vi "GSwFormDSP_Create.vi"(0 "reference in":refnum<class "GSwFormDSP.lvclass">, 5 "error in (no error)":errorcluster, 7 "Application Name":string, 9 "State Queue":string[](array[string])) -> (14 "reference out":refnum<class "GSwFormDSP.lvclass">, 19 "error out":errorcluster)   [LabVIEW 2020, in "GSwFormDSP.lvclass"]
doc: "Constructor."
uses:
  GSwFormDSP.lvclass
  C:/Program Files/National Instruments/LabVIEW 2020/vi.lib/addons/_AddQ/G#Object/G#Object.lvclass
  C:/Users/fcharett/docsWork/coding/20SPWB/C/Users/fcharett/docsWork/coding/LabVIEW/API/Generic Utilities_class/Generic Utilities.lvclass
  functions/TDF Parameters.ctl
  <vilib>/addons/_AddQ/G#Object/G#Object.lvclass
  Generic Utilities_class/Generic Utilities.lvclass
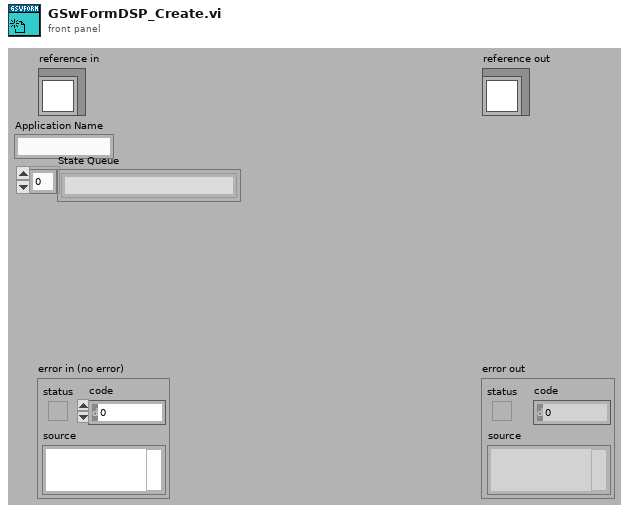
[diagram p1: front panel]
types:
  T1 = typedef "GSwFormDSP.lvclass/TDF Parameters.ctl" = cluster{"Filter":enum32{"Lowpass", "Highpass", "Bandpass", "Bandstop"}, "Type:":enum16{"Butterworth", "Chebyshev", "Inv Chebyshev", "Elliptic", "Bessel"}, "LP cutoff freq":dbl, "HP cutoff freq":dbl, "Order":i32, "passband ripple (dB)":dbl, "stopband attenuation (dB)":dbl, "Phaseless Filter":bool, "Include Fade IN and OUT":bool}
  T2 = typedef "GSwFormDSP.lvclass/ObjectAttributesRef.ctl" = refnum<data-value>
  T3 = typedef "GSwFormDSP.lvclass/ObjectAttributes.ctl" = cluster{"Wform Ref":refnum<data-value>, "Nb Signals":i32, "Spectral Function Parameters":T4, "FFT":waveform(cdb)[], "Nb FFT":i32, "Nb Averages":i32[], "Reference Indexes":i32[], "Response Indexes":i32[], "Coherence":waveform(dbl)[], "TDF Parameters":T1, "DAQ":cluster{"Duration (sec)":dbl, "Buffer Size (Samples)":i32, "Offset (Samples)":i32}, "Filter Impulse Response (TDF)":waveform(dbl), "Sound Playback":T6}
  T4 = typedef "GSwFormDSP.lvclass/Spectral Parameters.ctl" = cluster{"Frequency resolution (Hz)":dbl, "Overlap":dbl, "Window":T5}
  T5 = typedef "NI_AALPro.lvlib/windowTd.ctl" = u32
  T6 = typedef "GSwFormDSP.lvclass/Sound Playback.ctl" = cluster{"Timer start (ms)":u32, "task ID":T7, "Cursor Init Location (s)":dbl, "SC Volume":dbl}
  T7 = typedef "Sound Output Task ID.ctl" = u32
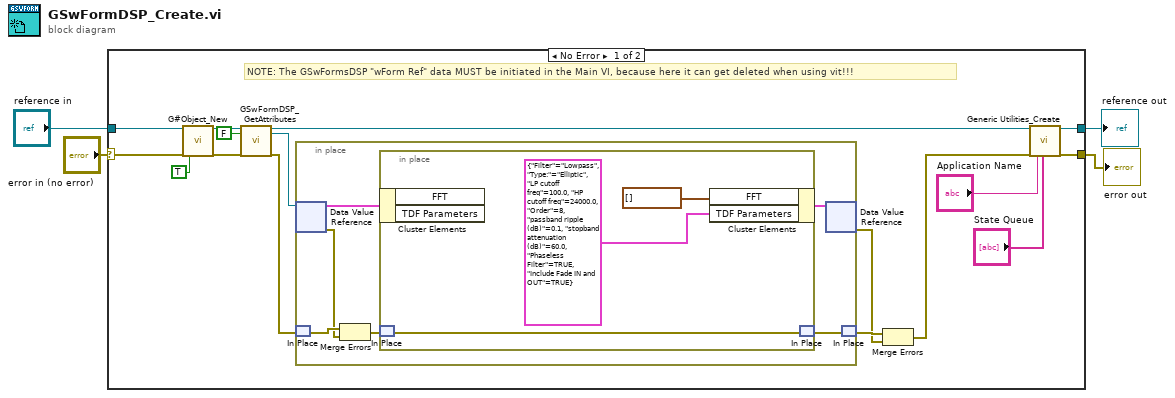
[diagram p0: block diagram]
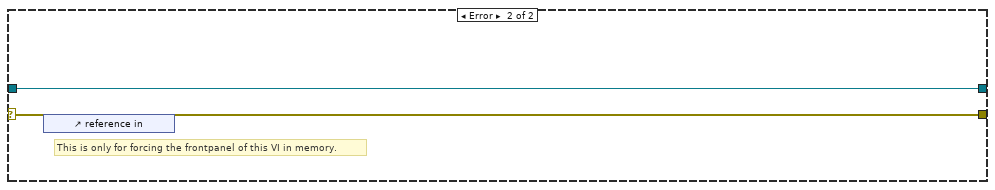
[diagram p2: hidden frame]
diagram:
  n1 = case shown="No Error" "error in (no error)" {
    selector: "error in (no error)" -> [w8 w31]
    tunnel: [w14 w31] -> w3
    tunnel: [w13 w30] -> w1
    tunnel: "reference in" -> [w7 w30]
    frame No Error {
      # "NOTE: The GSwFormsDSP \"wForm Ref\" data MUST be initiated in the Main VI, because here it can get deleted when using vit!!!"
      n2 = call <vilib>:"G#Object_New.vi"("reference in"=w7, "error in (no error)"=w8, "user counter (T)?"=TRUE ("User Counter")) -> ("reference out"=w19:refnum<class "GSwFormDSP.lvclass">, "error out"=w18:errorcluster)  [unwired: 14 in, 1 out]
      n3 = call "GSwFormDSP_GetAttributes.vi"("reference in"=w19, "return data? (T)"=FALSE, "error in (no error)"=w18) -> ("reference out"=w9:refnum<class "GSwFormDSP.lvclass">, "attributes ref"=w16:T2, "error out"=w12:errorcluster)  [unwired: 13 in, 1 out]
      n4 = in-place {
        n5 = in-place-dvr #1(w16) -> (w25:T3, w23:errorcluster)
        n6 = in-place-match #2(w12) -> (w24:errorcluster)
        n7 = Merge Errors(w24, w23) -> (w22:errorcluster)
        n8 = in-place {
          n9 = in-place-cluster #3(w25) -> ()  [unwired: 2 out]
          n10 = in-place-match #4(w22) -> (w27:errorcluster)
          n11 = in-place-cluster #3("FFT"=waveform(cdb)[] [], "TDF Parameters"=T1 {"Filter"=enum."Lowpass", "Type:"=enum."Elliptic", "LP cutoff freq"=100.0, "HP cutoff freq"=24000.0, "Order"=8, "passband ripple (dB)"=0.1, "stopband attenuation (dB)"=60.0, "Phaseless Filter"=TRUE, "Include Fade IN and OUT"=TRUE}) -> (w26:T3)
          n12 = in-place-match #4(w27) -> (w21:errorcluster)
        }
        n13 = in-place-dvr #1(w26) -> (w10:errorcluster)  [unwired: 1 out]
        n14 = in-place-match #2(w21) -> (w11:errorcluster)
      }
      n15 = Merge Errors(w11, w10) -> (w15:errorcluster)
      n16 = call "Generic Utilities_Create.vi"("reference in"=w9, "error in (no error)"=w15, "Application Name"="Application Name", "State Queue"="State Queue") -> ("reference out"=w13:refnum<class "GSwFormDSP.lvclass">, "error out"=w14:errorcluster)  [unwired: 14 in]
    }
    frame Error {
      # "This is only for forcing the frontpanel of this VI in memory."
      n17 = control-ref of="reference in"() -> ()  [unwired: 1 out]
    }
  }
  "error out" <- w3
  "reference out" <- w1
